vi "PH_ForceSensor.ProcCases.vi"(0 "i ref in":refnum<vi>, 1 "selector":string, 2 "Data":T1, 3 "call cluster":T2={"Object"="", "Selector"="", "CallType"=enum."synchronous", "Async Object"="", "Async Selector"="", "Data Descriptor"="", "Data"=[], "Error #"=0, "Expire"=0}, 5 "error in (no error)":errorcluster) -> (14 "i ref out":refnum<vi>, 17 "answer cluster":T2={"Object"="", "Selector"="", "CallType"=enum."synchronous", "Async Object"="", "Async Selector"="", "Data Descriptor"="", "Data"=[], "Error #"=0, "Expire"=0}, 19 "error out":errorcluster)   [LabVIEW 2014, in "PH_ForceSensor.lvlib"]
doc: "This method is called by a process from within the default case in the event loop. The methods of a class that are linked to events will be called from THIS method. Add your code here."
uses:
  PH_ForceSensor.lvlib
  CS_Core/CSSystem/CoreDefs/CoreDefs.call_type.ctl
  CS_Core/BaseProcess/BaseProcess.descriptor string definition.ctl
  CS_Core/CSSystem/CoreDefs/CoreDefs.rawDataType.ctl
  PH_Devices/PH_Beckhoff_StepMot/PH_Beckhoff_StepMot.Force Sensor Tags.ctl
  PH_Devices/PH_Beckhoff_StepMot/PH_Beckhoff_StepMot.Force Sensor Location.ctl
  PH_ForceSensor.Dataset.ctl
  PH_ForceSensor.Ranges.ctl
  CS_Core/CSSystem/CoreLib/CoreLib.string 2 byte array.vi
  CS_Core/CSSystem/CoreLib/CoreLib.byte array 2 double.vi
  CS_Core/BaseProcess/BaseProcess.lvlib
  CS_Core/CAEObj/CAEObj.lvlib
  CS_Core/CSSystem/CoreLib/CoreLib.lvlib
  PH_Basics/PH_PSDBWriter/PH_PSDBWriter.lvlib
  PH_Basics/PH_Common/PH_Common.lvlib
  PH_Devices/PH_Beckhoff_StepMot/PH_Beckhoff_StepMot.lvlib
  PHELIX/PH_BeamlineInformation/PH_BeamlineInformation.lvlib
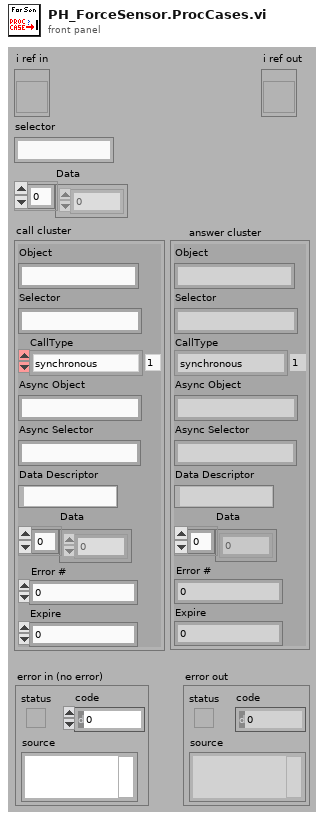
[diagram p1: front panel]
types:
  T1 = typedef "CoreDefs.rawDataType.ctl" = i8[]
  T2 = typedef "CoreDefs.call_type.ctl" = cluster{"Object":string, "Selector":string, "CallType":enum16{"simple", "synchronous", "asynchronous"}, "Async Object":string, "Async Selector":string, "Data Descriptor":T3, "Data":T1, "Error #":i32, "Expire":u32}
  T3 = typedef "BaseProcess.lvlib/BaseProcess.descriptor string definition.ctl" = string
  T4 = typedef "PH_Beckhoff_StepMot.lvlib/PH_Beckhoff_StepMot.Force Sensor Location.ctl" = enum16{"no Info", "MM1"}
  T5 = typedef "PH_ForceSensor.lvlib/PH_ForceSensor.Dataset.ctl" = cluster{"top front":dbl, "top back":dbl, "bottom front":dbl, "bottom back":dbl}
  T6 = typedef "PH_ForceSensor.lvlib/PH_ForceSensor.Ranges.ctl" = cluster{"Low Energy":cluster{"Upper Limit":dbl, "Lower Limit":dbl}, "High Energy":cluster{"Upper Limit":dbl, "Lower Limit":dbl}}
  T7 = typedef "PH_ForceSensor.lvlib/PH_ForceSensor.i attribute.ctl" = cluster{"GUI Refs":T8, "Rawvalues":T5, "Offsets [µV]":T5, "Scalings [mV/V]":T5, "Forces [N]":T5, "Supply Voltage [V]":dbl, "Full Force [N]":dbl, "Ranges [N]":cluster{"Low Energy":cluster{"Upper Limit":dbl, "Lower Limit":dbl}, "High Energy":cluster{"Upper Limit":dbl, "Lower Limit":dbl}}}
  T8 = typedef "PH_ForceSensor.lvlib/PH_ForceSensor.GUI Refs.ctl" = cluster{"Delete":refnum<vi>, "Rawvalues":refnum<vi>, "Offsets [µV]":refnum<vi>, "Sensor Values [µV]":refnum<vi>, "Scalings [mV/V]":refnum<vi>, "Supply Voltage [V]":refnum<vi>, "Full Force [N]":refnum<vi>, "Forces [N]":refnum<vi>, "Graph Differential Forces":refnum<vi>, "Graph Absolute Forces":refnum<vi>, "Ranges [N]":refnum<vi>}
  T9 = typedef "PH_Beckhoff_StepMot.lvlib/PH_Beckhoff_StepMot.Force Sensor Tags.ctl" = enum16{"top-front", "top-back", "bottom-front", "bottom-back"}
  T10 = typedef "PH_PSDBWriter.lvlib/PH_PSDBWriter.PHELIX-Subsystems.ctl" = i32
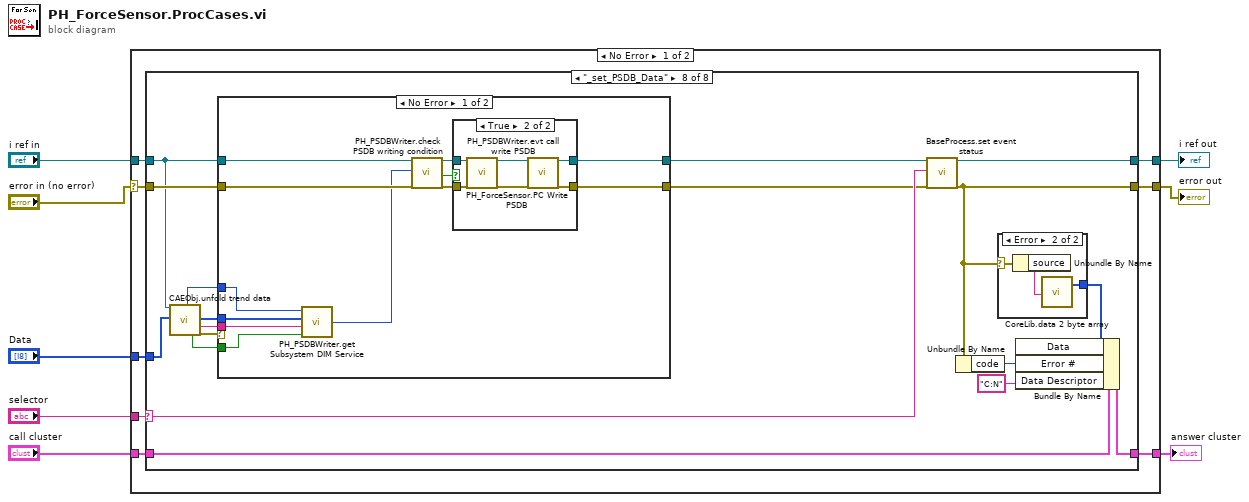
[diagram p0: block diagram]
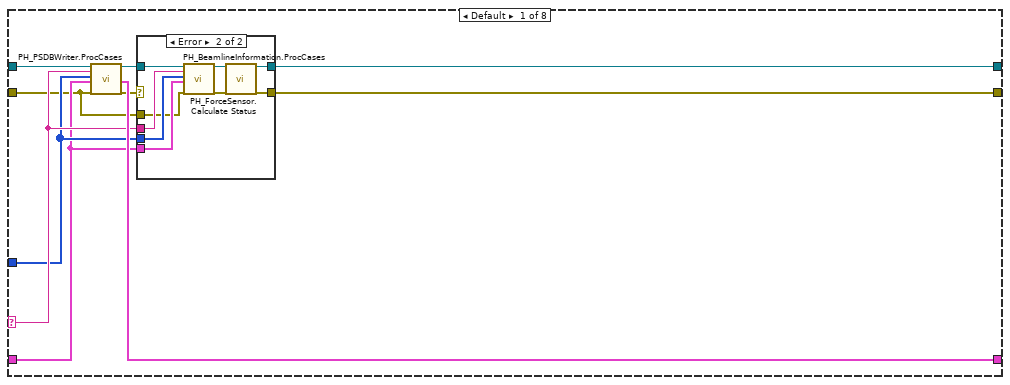
[diagram p2: hidden frame]
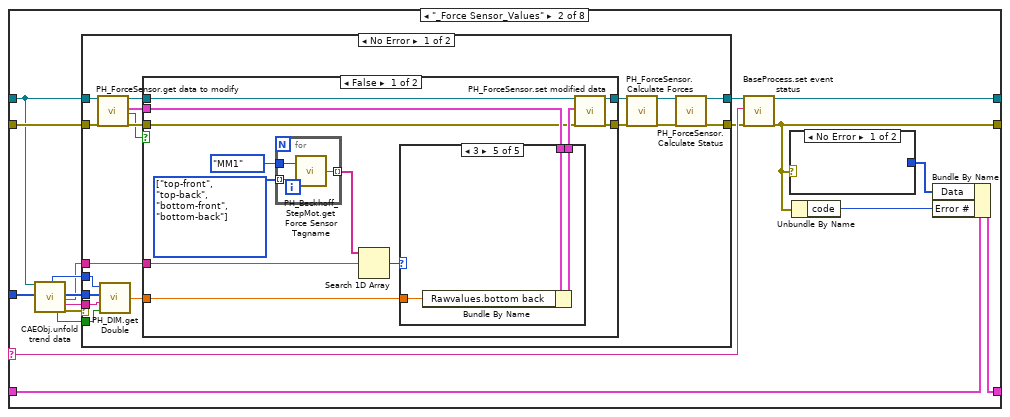
[diagram p4: hidden frame]
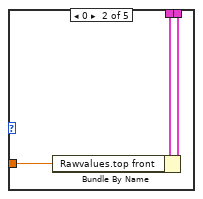
[diagram p6: hidden frame]
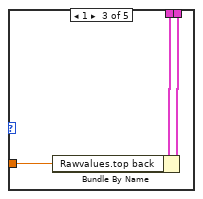
[diagram p7: hidden frame]
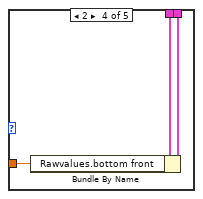
[diagram p8: hidden frame]
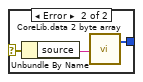
[diagram p11: hidden frame]
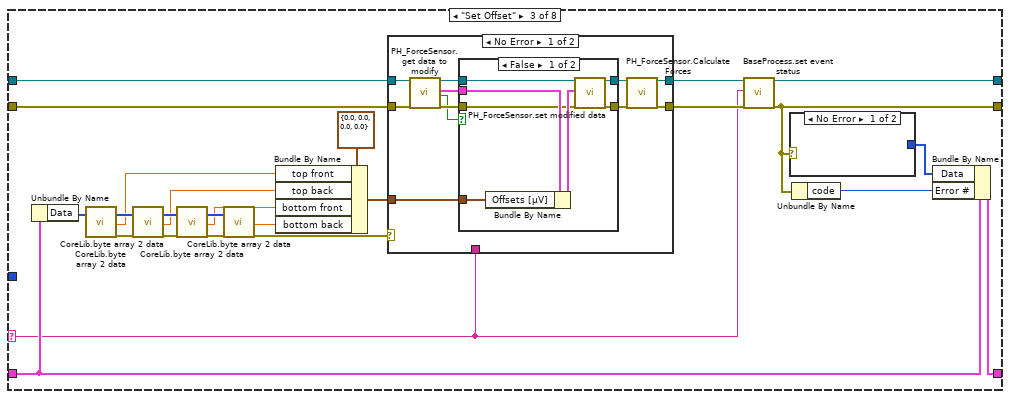
[diagram p12: hidden frame]
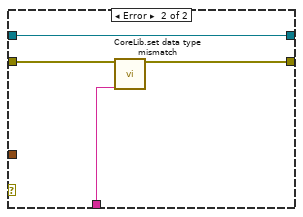
[diagram p14: hidden frame]
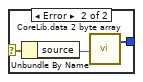
[diagram p15: hidden frame]
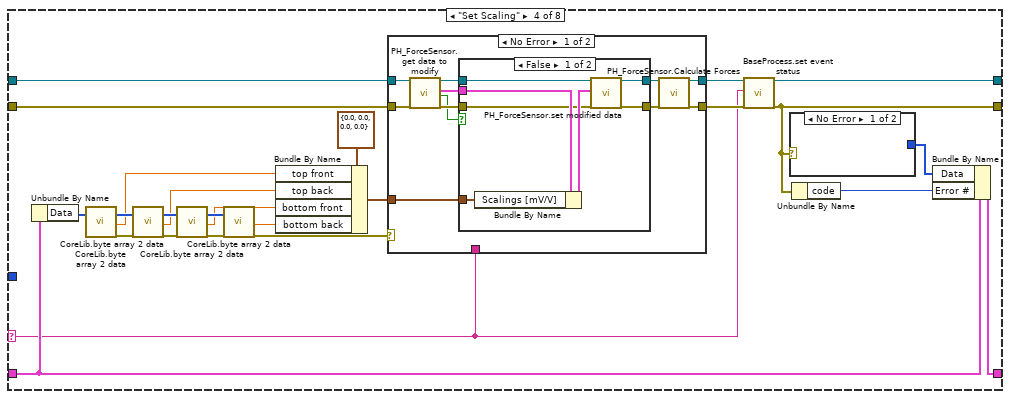
[diagram p16: hidden frame]
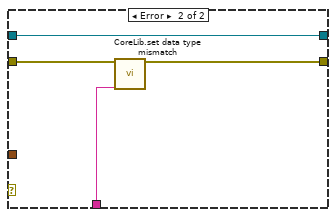
[diagram p18: hidden frame]
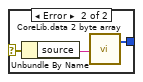
[diagram p19: hidden frame]
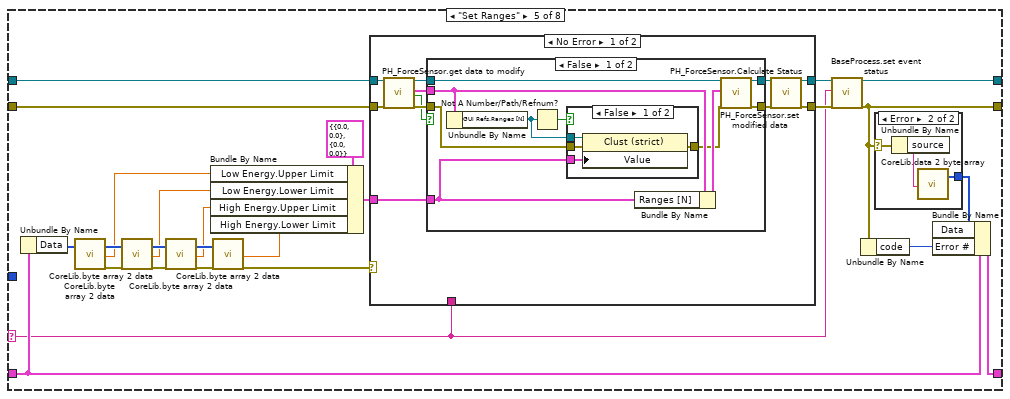
[diagram p20: hidden frame]
diagram:
  n1 = case shown="No Error" "error in (no error)" {
    selector: "error in (no error)" -> [w9 w400]
    tunnel: "selector" -> [w16 _]
    tunnel: [w15 w399] -> w7
    tunnel: "call cluster" -> [w14 w399]
    tunnel: "i ref in" -> [w13 w401]
    tunnel: [w12 w401] -> w4
    tunnel: [w11 w400] -> w3
    tunnel: "Data" -> [w10 _]
    frame No Error {
      n2 = case shown="\"_set_PSDB_Data\"" w16 {
        selector: w16 -> [w20 w50 w109 w161 w213 w275 w316 w365]
        tunnel: w10 -> [w19 w41 _ _ _ _ _ w361]
        tunnel: w13 -> [w25 w40 w125 w177 w229 w278 w319 w360]
        tunnel: [w22 w53 w131 w183 w235 w284 w325 w367] -> w12
        tunnel: w14 -> [w18 w49 w123 w175 w227 w276 w317 w362]
        tunnel: [w26 w51 w129 w181 w233 w282 w323 w364] -> w15
        tunnel: w9 -> [w17 w48 w128 w180 w232 w281 w322 w372]
        tunnel: [w24 w52 w130 w182 w234 w283 w324 w366] -> w11
        frame Default {
          n3 = call "PH_PSDBWriter.ProcCases.vi"("i ref in"=w25, "selector"=w20, "Data"=w19, "call cluster"=w18, "error in"=w17) -> ("i ref out"=w23:refnum<vi>, "answer cluster"=w26:T2, "error out"=w21:errorcluster)  [unwired: 12 in]
          n4 = case shown="Error" w21 {
            selector: w21 -> [w27 _]
            tunnel: [w27 w32] -> w24
            tunnel: w23 -> [w28 w36]
            tunnel: [w28 w30] -> w22
            tunnel: w20 -> [_ w35]
            tunnel: w19 -> [_ w34]
            tunnel: w18 -> [_ w33]
            tunnel: w17 -> [_ w29]
            frame No Error {
            }
            frame Error {
              n5 = call "PH_BeamlineInformation.ProcCases.vi"("i ref in"=w36, "selector"=w35, "Data"=w34, "call cluster"=w33, "error in (no error)"=w29) -> ("i ref out"=w31:refnum<vi>, "error out"=w37:errorcluster)  [unwired: 12 in, 1 out]
              n6 = call "PH_ForceSensor.Calculate Status.vi"("VI in"=w31, "error in"=w37) -> ("VI out"=w30:refnum<vi>, "error out"=w32:errorcluster)  [unwired: 16 in]
            }
          }
        }
        frame "_Force Sensor_Values" {
          n7 = call "CAEObj.unfold trend data.vi"("i ref in"=w40, "raw trend data"=w41) -> ("quality"=w43:i32, "no link"=w42:bool, "data"=w45:i8[], "serviceName"=w38:string, "typeDescriptor"=w39:string, "error out"=w44:errorcluster)  [unwired: 9 in, 3 out]
          n8 = case shown="No Error" w44 {
            tunnel: [w56 w105] -> w47
            tunnel: [w58 w104] -> w46
            tunnel: w39 -> [w73 _]
            tunnel: w45 -> [w72 _]
            tunnel: w43 -> [w71 _]
            tunnel: w42 -> [w70 _]
            tunnel: w40 -> [w68 w105]
            tunnel: w48 -> [w69 w104]
            tunnel: w38 -> [w61 _]
            frame No Error {
              n9 = call "PH_ForceSensor.get data to modify.vi"("i ref in"=w68, "error in (no error)"=w69) -> ("i ref out"=w67:refnum<vi>, "i attribute"=w64:T7, "timed out"=w63:bool, "error out"=w66:errorcluster)  [unwired: 14 in]
              n10 = call "PH_DIM.get Double.vi"("no link"=w70, "typeDescriptor"=w73, "data"=w72, "quality"=w71) -> ("Value"=w62:dbl)
              n11 = case shown="False" w63 {
                tunnel: w67 -> [w85 w103]
                tunnel: [w84 w103] -> w59
                tunnel: w66 -> [w75 w102]
                tunnel: [w83 w102] -> w65
                tunnel: w64 -> [w82 _]
                tunnel: w62 -> [w80 _]
                tunnel: w61 -> [w76 _]
                frame False {
                  w78 = T9[] [enum."top-front", enum."top-back", enum."bottom-front", enum."bottom-back"] items=["top-front", "top-back", "bottom-front", "bottom-back"]
                  n12 = for {
                    tunnel: PH_Beckhoff_StepMot.Force_Sensor_Location."MM1" ("Force Sensor Location") -> [w101]
                    tunnel: w78 -> [w100] mode=indexing
                    tunnel: [w99] -> w79 mode=indexing
                    n13 = call "PH_Beckhoff_StepMot.get Force Sensor Tagname.vi"("Force Sensor Tag"=w100, "Force Sensor Location"=w101) -> ("Force Sensor Tagname"=w99:string)
                  }
                  n14 = Search 1D Array(1D array=w79, element=w76) -> (index of element=w74:i32)  [unwired: 1 in]
                  n15 = case shown="3" w74 {
                    tunnel: w82 -> [w86 w89 w92 w95 w98]
                    tunnel: [w86 w88 w91 w94 w97] -> w81
                    tunnel: w80 -> [_ w87 w90 w93 w96]
                    frame Default {
                    }
                    frame 0 {
                      n16 = Bundle By Name(cluster=w89, "Rawvalues.top front"=w87) -> (w88:T7)
                    }
                    frame 1 {
                      n17 = Bundle By Name(cluster=w92, "Rawvalues.top back"=w90) -> (w91:T7)
                    }
                    frame 2 {
                      n18 = Bundle By Name(cluster=w95, "Rawvalues.bottom front"=w93) -> (w94:T7)
                    }
                    frame 3 {
                      n19 = Bundle By Name(cluster=w98, "Rawvalues.bottom back"=w96) -> (w97:T7)
                    }
                  }
                  n20 = call "PH_ForceSensor.set modified data.vi"("i ref in"=w85, "i attribute"=w81, "error in (no error)"=w75) -> ("i ref out"=w84:refnum<vi>, "error out"=w83:errorcluster)  [unwired: 15 in]
                }
                frame True {
                }
              }
              n21 = call "PH_ForceSensor.Calculate Forces.vi"("VI in"=w59, "error in"=w65) -> ("VI out"=w57:refnum<vi>, "error out"=w60:errorcluster)  [unwired: 16 in]
              n22 = call "PH_ForceSensor.Calculate Status.vi"("VI in"=w57, "error in"=w60) -> ("VI out"=w56:refnum<vi>, "error out"=w58:errorcluster)  [unwired: 16 in]
            }
            frame Error {
            }
          }
          n23 = call "BaseProcess.set event status.vi"("i ref in"=w47, "EventStatus"=w50, "error in (no error)"=w46) -> ("i ref out"=w53:refnum<vi>, "error out"=w52:errorcluster)  [unwired: 14 in, 1 out]
          n24 = case shown="No Error" w52 {
            selector: w52 -> [_ w108]
            tunnel: [_ w106] -> w54
            frame No Error {
            }
            frame Error {
              n25 = Unbundle By Name(w108) -> ("source"=w107:string)
              n26 = call-poly "CoreLib.data 2 byte array.vi"("string"=w107) -> ("byteArray out"=w106:T1)  [unwired: 18 in]
            }
          }
          n27 = Unbundle By Name(w52) -> ("code"=w55:i32)
          n28 = Bundle By Name(cluster=w49, "Data"=w54, "Error #"=w55) -> (w51:T2)
        }
        frame "Set Offset" {
          n29 = Unbundle By Name(w123) -> ("Data"=w124:T1)
          n30 = call-poly "CoreLib.byte array 2 data.vi"("byteArray"=w124) -> ("byteArray out"=w119:T1, "d64"=w114:dbl, "error out"=w122:errorcluster)  [unwired: 16 in]
          n31 = call-poly "CoreLib.byte array 2 data.vi"("byteArray"=w119, "error in (no error)"=w122) -> ("byteArray out"=w118:T1, "d64"=w113:dbl, "error out"=w121:errorcluster)  [unwired: 15 in]
          n32 = call-poly "CoreLib.byte array 2 data.vi"("byteArray"=w118, "error in (no error)"=w121) -> ("byteArray out"=w117:T1, "d64"=w112:dbl, "error out"=w120:errorcluster)  [unwired: 15 in]
          n33 = call-poly "CoreLib.byte array 2 data.vi"("byteArray"=w117, "error in (no error)"=w120) -> ("d64"=w111:dbl, "error out"=w116:errorcluster)  [unwired: 15 in, 1 out]
          n34 = Bundle By Name(cluster=T5 {"top front"=0.0, "top back"=0.0, "bottom front"=0.0, "bottom back"=0.0} ("Dataset"), "top front"=w114, "top back"=w113, "bottom front"=w112, "bottom back"=w111) -> (w110:T5)
          n35 = case shown="No Error" w116 {
            tunnel: [w135 w157] -> w127
            tunnel: [w137 w155] -> w126
            tunnel: w125 -> [w143 w157]
            tunnel: w128 -> [w144 w156]
            tunnel: w110 -> [w134 _]
            tunnel: w109 -> [_ w154]
            frame No Error {
              n36 = call "PH_ForceSensor.get data to modify.vi"("i ref in"=w143, "error in (no error)"=w144) -> ("i ref out"=w142:refnum<vi>, "i attribute"=w139:T7, "timed out"=w138:bool, "error out"=w141:errorcluster)  [unwired: 14 in]
              n37 = case shown="False" w138 {
                tunnel: w142 -> [w151 w153]
                tunnel: [w150 w153] -> w136
                tunnel: w141 -> [w146 w152]
                tunnel: [w149 w152] -> w140
                tunnel: w139 -> [w148 _]
                tunnel: w134 -> [w145 _]
                frame False {
                  n38 = Bundle By Name(cluster=w148, "Offsets [µV]"=w145) -> (w147:T7)
                  n39 = call "PH_ForceSensor.set modified data.vi"("i ref in"=w151, "i attribute"=w147, "error in (no error)"=w146) -> ("i ref out"=w150:refnum<vi>, "error out"=w149:errorcluster)  [unwired: 15 in]
                }
                frame True {
                }
              }
              n40 = call "PH_ForceSensor.Calculate Forces.vi"("VI in"=w136, "error in"=w140) -> ("VI out"=w135:refnum<vi>, "error out"=w137:errorcluster)  [unwired: 16 in]
            }
            frame Error {
              n41 = call "CoreLib.set data type mismatch.vi"("error in (no error)"=w156, "error source"=w154) -> ("error out"=w155:errorcluster)  [unwired: 17 in]
            }
          }
          n42 = call "BaseProcess.set event status.vi"("i ref in"=w127, "EventStatus"=w109, "error in (no error)"=w126) -> ("i ref out"=w131:refnum<vi>, "error out"=w130:errorcluster)  [unwired: 14 in, 1 out]
          n43 = case shown="No Error" w130 {
            selector: w130 -> [_ w160]
            tunnel: [_ w158] -> w132
            frame No Error {
            }
            frame Error {
              n44 = Unbundle By Name(w160) -> ("source"=w159:string)
              n45 = call-poly "CoreLib.data 2 byte array.vi"("string"=w159) -> ("byteArray out"=w158:T1)  [unwired: 18 in]
            }
          }
          n46 = Unbundle By Name(w130) -> ("code"=w133:i32)
          n47 = Bundle By Name(cluster=w123, "Data"=w132, "Error #"=w133) -> (w129:T2)
        }
        frame "Set Scaling" {
          n48 = Unbundle By Name(w175) -> ("Data"=w176:T1)
          n49 = call-poly "CoreLib.byte array 2 data.vi"("byteArray"=w176) -> ("byteArray out"=w171:T1, "d64"=w166:dbl, "error out"=w174:errorcluster)  [unwired: 16 in]
          n50 = call-poly "CoreLib.byte array 2 data.vi"("byteArray"=w171, "error in (no error)"=w174) -> ("byteArray out"=w170:T1, "d64"=w165:dbl, "error out"=w173:errorcluster)  [unwired: 15 in]
          n51 = call-poly "CoreLib.byte array 2 data.vi"("byteArray"=w170, "error in (no error)"=w173) -> ("byteArray out"=w169:T1, "d64"=w164:dbl, "error out"=w172:errorcluster)  [unwired: 15 in]
          n52 = call-poly "CoreLib.byte array 2 data.vi"("byteArray"=w169, "error in (no error)"=w172) -> ("d64"=w163:dbl, "error out"=w168:errorcluster)  [unwired: 15 in, 1 out]
          n53 = Bundle By Name(cluster=T5 {"top front"=0.0, "top back"=0.0, "bottom front"=0.0, "bottom back"=0.0} ("Dataset"), "top front"=w166, "top back"=w165, "bottom front"=w164, "bottom back"=w163) -> (w162:T5)
          n54 = case shown="No Error" w168 {
            tunnel: [w187 w209] -> w179
            tunnel: [w189 w207] -> w178
            tunnel: w177 -> [w195 w209]
            tunnel: w180 -> [w196 w208]
            tunnel: w162 -> [w186 _]
            tunnel: w161 -> [_ w206]
            frame No Error {
              n55 = call "PH_ForceSensor.get data to modify.vi"("i ref in"=w195, "error in (no error)"=w196) -> ("i ref out"=w194:refnum<vi>, "i attribute"=w191:T7, "timed out"=w190:bool, "error out"=w193:errorcluster)  [unwired: 14 in]
              n56 = case shown="False" w190 {
                tunnel: w194 -> [w203 w205]
                tunnel: [w202 w205] -> w188
                tunnel: w193 -> [w198 w204]
                tunnel: [w201 w204] -> w192
                tunnel: w191 -> [w200 _]
                tunnel: w186 -> [w197 _]
                frame False {
                  n57 = Bundle By Name(cluster=w200, "Scalings [mV/V]"=w197) -> (w199:T7)
                  n58 = call "PH_ForceSensor.set modified data.vi"("i ref in"=w203, "i attribute"=w199, "error in (no error)"=w198) -> ("i ref out"=w202:refnum<vi>, "error out"=w201:errorcluster)  [unwired: 15 in]
                }
                frame True {
                }
              }
              n59 = call "PH_ForceSensor.Calculate Forces.vi"("VI in"=w188, "error in"=w192) -> ("VI out"=w187:refnum<vi>, "error out"=w189:errorcluster)  [unwired: 16 in]
            }
            frame Error {
              n60 = call "CoreLib.set data type mismatch.vi"("error in (no error)"=w208, "error source"=w206) -> ("error out"=w207:errorcluster)  [unwired: 17 in]
            }
          }
          n61 = call "BaseProcess.set event status.vi"("i ref in"=w179, "EventStatus"=w161, "error in (no error)"=w178) -> ("i ref out"=w183:refnum<vi>, "error out"=w182:errorcluster)  [unwired: 14 in, 1 out]
          n62 = case shown="No Error" w182 {
            selector: w182 -> [_ w212]
            tunnel: [_ w210] -> w184
            frame No Error {
            }
            frame Error {
              n63 = Unbundle By Name(w212) -> ("source"=w211:string)
              n64 = call-poly "CoreLib.data 2 byte array.vi"("string"=w211) -> ("byteArray out"=w210:T1)  [unwired: 18 in]
            }
          }
          n65 = Unbundle By Name(w182) -> ("code"=w185:i32)
          n66 = Bundle By Name(cluster=w175, "Data"=w184, "Error #"=w185) -> (w181:T2)
        }
        frame "Set Ranges" {
          n67 = Unbundle By Name(w227) -> ("Data"=w228:T1)
          n68 = call-poly "CoreLib.byte array 2 data.vi"("byteArray"=w228) -> ("byteArray out"=w223:T1, "d64"=w218:dbl, "error out"=w226:errorcluster)  [unwired: 16 in]
          n69 = call-poly "CoreLib.byte array 2 data.vi"("byteArray"=w223, "error in (no error)"=w226) -> ("byteArray out"=w222:T1, "d64"=w217:dbl, "error out"=w225:errorcluster)  [unwired: 15 in]
          n70 = call-poly "CoreLib.byte array 2 data.vi"("byteArray"=w222, "error in (no error)"=w225) -> ("byteArray out"=w221:T1, "d64"=w216:dbl, "error out"=w224:errorcluster)  [unwired: 15 in]
          n71 = call-poly "CoreLib.byte array 2 data.vi"("byteArray"=w221, "error in (no error)"=w224) -> ("d64"=w215:dbl, "error out"=w220:errorcluster)  [unwired: 15 in, 1 out]
          n72 = Bundle By Name(cluster=T6 {"Low Energy"={"Upper Limit"=0.0, "Lower Limit"=0.0}, "High Energy"={"Upper Limit"=0.0, "Lower Limit"=0.0}} ("Ranges [N]"), "Low Energy.Upper Limit"=w218, "Low Energy.Lower Limit"=w217, "High Energy.Upper Limit"=w216, "High Energy.Lower Limit"=w215) -> (w214:T6)
          n73 = case shown="No Error" w220 {
            tunnel: [w239 w269] -> w231
            tunnel: [w241 w267] -> w230
            tunnel: w229 -> [w247 w269]
            tunnel: w232 -> [w248 w268]
            tunnel: w214 -> [w238 _]
            tunnel: w213 -> [_ w266]
            frame No Error {
              n74 = call "PH_ForceSensor.get data to modify.vi"("i ref in"=w247, "error in (no error)"=w248) -> ("i ref out"=w246:refnum<vi>, "i attribute"=w243:T7, "timed out"=w242:bool, "error out"=w245:errorcluster)  [unwired: 14 in]
              n75 = case shown="False" w242 {
                tunnel: w246 -> [w258 w265]
                tunnel: [w257 w265] -> w240
                tunnel: w245 -> [w254 w264]
                tunnel: [w256 w264] -> w244
                tunnel: w243 -> [w253 _]
                tunnel: w238 -> [w251 _]
                frame False {
                  n76 = Unbundle By Name(w253) -> ("GUI Refs.Ranges [N]"=w249:refnum<vi>)
                  n77 = Not A Number/Path/Refnum?(number/path/refnum=w249) -> (NaN/Path/Refnum?=w250:bool)
                  n78 = case shown="False" w250 {
                    tunnel: w254 -> [w262 w263]
                    tunnel: [w261 w263] -> w252
                    tunnel: w249 -> [w260 _]
                    tunnel: w251 -> [w259 _]
                    frame False {
                      n79 = property class="Clust (strict)"(reference=w260, error in=w262, "Value"=w259) -> (error out=w261:errorcluster)  [unwired: 1 out]
                    }
                    frame True {
                    }
                  }
                  n80 = Bundle By Name(cluster=w253, "Ranges [N]"=w251) -> (w255:T7)
                  n81 = call "PH_ForceSensor.set modified data.vi"("i ref in"=w258, "i attribute"=w255, "error in (no error)"=w252) -> ("i ref out"=w257:refnum<vi>, "error out"=w256:errorcluster)  [unwired: 15 in]
                }
                frame True {
                }
              }
              n82 = call "PH_ForceSensor.Calculate Status.vi"("VI in"=w240, "error in"=w244) -> ("VI out"=w239:refnum<vi>, "error out"=w241:errorcluster)  [unwired: 16 in]
            }
            frame Error {
              n83 = call "CoreLib.set data type mismatch.vi"("error in (no error)"=w268, "error source"=w266) -> ("error out"=w267:errorcluster)  [unwired: 17 in]
            }
          }
          n84 = call "BaseProcess.set event status.vi"("i ref in"=w231, "EventStatus"=w213, "error in (no error)"=w230) -> ("i ref out"=w235:refnum<vi>, "error out"=w234:errorcluster)  [unwired: 14 in, 1 out]
          n85 = Unbundle By Name(w234) -> ("code"=w237:i32)
          n86 = case shown="Error" w234 {
            selector: w234 -> [_ w272]
            tunnel: [_ w270] -> w236
            frame No Error {
            }
            frame Error {
              n87 = Unbundle By Name(w272) -> ("source"=w271:string)
              n88 = call-poly "CoreLib.data 2 byte array.vi"("string"=w271) -> ("byteArray out"=w270:T1)  [unwired: 18 in]
            }
          }
          n89 = Bundle By Name(cluster=w227, "Data"=w236, "Error #"=w237) -> (w233:T2)
        }
        frame "Set Supply Voltage" {
          n90 = Unbundle By Name(w276) -> ("Data"=w277:T1)
          n91 = call-poly "CoreLib.byte array 2 data.vi"("byteArray"=w277) -> ("d64"=w274:dbl, "error out"=w273:errorcluster)  [unwired: 16 in, 1 out]
          n92 = case shown="No Error" w273 {
            tunnel: [w288 w310] -> w280
            tunnel: [w290 w308] -> w279
            tunnel: w278 -> [w296 w310]
            tunnel: w281 -> [w297 w309]
            tunnel: w274 -> [w287 _]
            tunnel: w275 -> [_ w307]
            frame No Error {
              n93 = call "PH_ForceSensor.get data to modify.vi"("i ref in"=w296, "error in (no error)"=w297) -> ("i ref out"=w295:refnum<vi>, "i attribute"=w292:T7, "timed out"=w291:bool, "error out"=w294:errorcluster)  [unwired: 14 in]
              n94 = case shown="False" w291 {
                tunnel: w295 -> [w304 w306]
                tunnel: [w303 w306] -> w289
                tunnel: w294 -> [w299 w305]
                tunnel: [w302 w305] -> w293
                tunnel: w292 -> [w301 _]
                tunnel: w287 -> [w298 _]
                frame False {
                  n95 = Bundle By Name(cluster=w301, "Supply Voltage [V]"=w298) -> (w300:T7)
                  n96 = call "PH_ForceSensor.set modified data.vi"("i ref in"=w304, "i attribute"=w300, "error in (no error)"=w299) -> ("i ref out"=w303:refnum<vi>, "error out"=w302:errorcluster)  [unwired: 15 in]
                }
                frame True {
                }
              }
              n97 = call "PH_ForceSensor.Calculate Forces.vi"("VI in"=w289, "error in"=w293) -> ("VI out"=w288:refnum<vi>, "error out"=w290:errorcluster)  [unwired: 16 in]
            }
            frame Error {
              n98 = call "CoreLib.set data type mismatch.vi"("error in (no error)"=w309, "error source"=w307) -> ("error out"=w308:errorcluster)  [unwired: 17 in]
            }
          }
          n99 = call "BaseProcess.set event status.vi"("i ref in"=w280, "EventStatus"=w275, "error in (no error)"=w279) -> ("i ref out"=w284:refnum<vi>, "error out"=w283:errorcluster)  [unwired: 14 in, 1 out]
          n100 = case shown="No Error" w283 {
            selector: w283 -> [_ w313]
            tunnel: [_ w311] -> w285
            frame No Error {
            }
            frame Error {
              n101 = Unbundle By Name(w313) -> ("source"=w312:string)
              n102 = call-poly "CoreLib.data 2 byte array.vi"("string"=w312) -> ("byteArray out"=w311:T1)  [unwired: 18 in]
            }
          }
          n103 = Unbundle By Name(w283) -> ("code"=w286:i32)
          n104 = Bundle By Name(cluster=w276, "Data"=w285, "Error #"=w286) -> (w282:T2)
        }
        frame "Set Full Force" {
          n105 = Unbundle By Name(w317) -> ("Data"=w318:T1)
          n106 = call-poly "CoreLib.byte array 2 data.vi"("byteArray"=w318) -> ("d64"=w315:dbl, "error out"=w314:errorcluster)  [unwired: 16 in, 1 out]
          n107 = case shown="No Error" w314 {
            tunnel: [w329 w351] -> w321
            tunnel: [w331 w349] -> w320
            tunnel: w319 -> [w337 w351]
            tunnel: w322 -> [w338 w350]
            tunnel: w315 -> [w328 _]
            tunnel: w316 -> [_ w348]
            frame No Error {
              n108 = call "PH_ForceSensor.get data to modify.vi"("i ref in"=w337, "error in (no error)"=w338) -> ("i ref out"=w336:refnum<vi>, "i attribute"=w333:T7, "timed out"=w332:bool, "error out"=w335:errorcluster)  [unwired: 14 in]
              n109 = case shown="False" w332 {
                tunnel: w336 -> [w345 w347]
                tunnel: [w344 w347] -> w330
                tunnel: w335 -> [w340 w346]
                tunnel: [w343 w346] -> w334
                tunnel: w333 -> [w342 _]
                tunnel: w328 -> [w339 _]
                frame False {
                  n110 = Bundle By Name(cluster=w342, "Full Force [N]"=w339) -> (w341:T7)
                  n111 = call "PH_ForceSensor.set modified data.vi"("i ref in"=w345, "i attribute"=w341, "error in (no error)"=w340) -> ("i ref out"=w344:refnum<vi>, "error out"=w343:errorcluster)  [unwired: 15 in]
                }
                frame True {
                }
              }
              n112 = call "PH_ForceSensor.Calculate Forces.vi"("VI in"=w330, "error in"=w334) -> ("VI out"=w329:refnum<vi>, "error out"=w331:errorcluster)  [unwired: 16 in]
            }
            frame Error {
              n113 = call "CoreLib.set data type mismatch.vi"("error in (no error)"=w350, "error source"=w348) -> ("error out"=w349:errorcluster)  [unwired: 17 in]
            }
          }
          n114 = call "BaseProcess.set event status.vi"("i ref in"=w321, "EventStatus"=w316, "error in (no error)"=w320) -> ("i ref out"=w325:refnum<vi>, "error out"=w324:errorcluster)  [unwired: 14 in, 1 out]
          n115 = case shown="No Error" w324 {
            selector: w324 -> [_ w354]
            tunnel: [_ w352] -> w326
            frame No Error {
            }
            frame Error {
              n116 = Unbundle By Name(w354) -> ("source"=w353:string)
              n117 = call-poly "CoreLib.data 2 byte array.vi"("string"=w353) -> ("byteArray out"=w352:T1)  [unwired: 18 in]
            }
          }
          n118 = Unbundle By Name(w324) -> ("code"=w327:i32)
          n119 = Bundle By Name(cluster=w317, "Data"=w326, "Error #"=w327) -> (w323:T2)
        }
        frame "_set_PSDB_Data" {
          n120 = call "CAEObj.unfold trend data.vi"("i ref in"=w360, "raw trend data"=w361) -> ("quality"=w355:i32, "no link"=w358:bool, "data"=w356:i8[], "typeDescriptor"=w357:string, "error out"=w359:errorcluster)  [unwired: 9 in, 4 out]
          n121 = case shown="No Error" w359 {
            tunnel: w372 -> [w384 w394]
            tunnel: [w383 w393] -> w368
            tunnel: [w382 w394] -> w363
            tunnel: w360 -> [w380 w393]
            tunnel: w358 -> [w375 _]
            tunnel: w357 -> [w374 _]
            tunnel: w356 -> [w377 _]
            tunnel: w355 -> [w376 _]
            frame No Error {
              n122 = call "PH_PSDBWriter.get Subsystem DIM Service.vi"("no link"=w375, "typeDescriptor"=w374, "data"=w377, "quality"=w376) -> ("PHELIX Subsystems"=w373:T10)
              n123 = call "PH_PSDBWriter.check PSDB writing condition.vi"("i ref in"=w380, "wanted Subsystem"=w373, "error IO"=w384) -> ("i ref out"=w379:refnum<vi>, "write PSDB?"=w378:bool, "error out"=w381:errorcluster)  [unwired: 14 in]
              n124 = case shown="True" w378 {
                tunnel: w381 -> [w385 w392]
                tunnel: [w386 w389] -> w383
                tunnel: [w385 w387] -> w382
                tunnel: w379 -> [w386 w391]
                frame False {
                }
                frame True {
                  n125 = call "PH_ForceSensor.PC Write PSDB.vi"("i ref in"=w391, "error IO"=w392) -> ("i ref out"=w390:refnum<vi>, "error out"=w388:errorcluster)  [unwired: 16 in]
                  n126 = call "PH_PSDBWriter.evt call write PSDB.vi"("i ref in"=w390, "error in (no error)"=w388) -> ("i ref out"=w389:refnum<vi>, "error out"=w387:errorcluster)  [unwired: 16 in]
                }
              }
            }
            frame Error {
            }
          }
          n127 = call "BaseProcess.set event status.vi"("i ref in"=w368, "EventStatus"=w365, "error in (no error)"=w363) -> ("i ref out"=w367:refnum<vi>, "error out"=w366:errorcluster)  [unwired: 14 in, 1 out]
          n128 = Unbundle By Name(w366) -> ("code"=w371:i32)
          n129 = case shown="Error" w366 {
            selector: w366 -> [_ w398]
            tunnel: [T1 [] ("byteArray out") w396] -> w369
            frame No Error {
            }
            frame Error {
              n130 = Unbundle By Name(w398) -> ("source"=w397:string)
              n131 = call-poly "CoreLib.data 2 byte array.vi"("string"=w397) -> ("byteArray out"=w396:T1)  [unwired: 18 in]
            }
          }
          n132 = Bundle By Name(cluster=w362, "Data"=w369, "Error #"=w371, "Data Descriptor"="C:N") -> (w364:T2)
        }
      }
    }
    frame Error {
    }
  }
  "answer cluster" <- w7
  "i ref out" <- w4
  "error out" <- w3
